vi "Set Control Value.vi"(8 "error in (no error)":errorcluster, 9 "value":variant, 11 "Panel":refnum<vi>) -> (0 "error out":errorcluster, 3 "Panel out":refnum<vi>)   [LabVIEW 2018, in "NISAST VI Scripting.lvlib" / "VI.lvlib" / "Front Panel.lvlib"]
uses:
  Front Panel.lvlib
  Type Define/Object Class.ctl
  Agilent N5232A PNA-L/Labview Driver/Keysight PNA Series/express/Utility/StudioHelper/Common/VI Scripting/Type Define/Type Define.lvlib
panel:
  in  "label":string
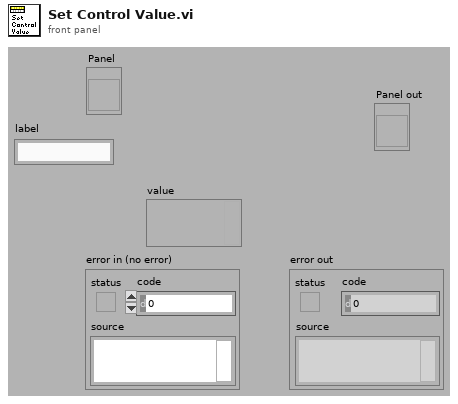
[diagram p1: front panel]
types:
  T1 = typedef "NISAST VI Scripting.lvlib/Type Define.lvlib/Object Class.ctl" = string
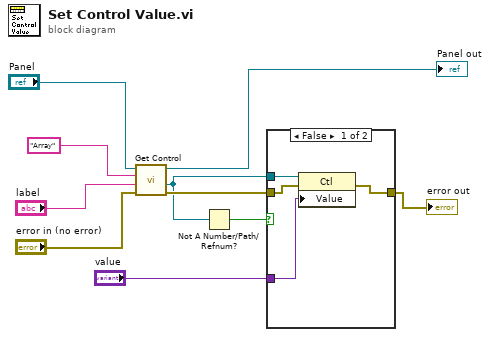
[diagram p0: block diagram]
diagram:
  n1 = call "Get Control.vi"("error in (no error)"="error in (no error)", "label"="label", "object class"=T1 "Array", "Panel"="Panel") -> ("error out"=w8:errorcluster, "first control"=w1:refnum<vi>, "Panel out"=→"Panel out":refnum<vi>)  [unwired: 5 out]
  n2 = Not A Number/Path/Refnum?(number/path/refnum=w1) -> (NaN/Path/Refnum?=w2:bool)
  n3 = case shown="False" w2 {
    tunnel: w1 -> [w14 _]
    tunnel: w8 -> [w13 w15]
    tunnel: "value" -> [w12 _]
    tunnel: [w11 w15] -> w5
    frame False {
      n4 = property class="Ctl"(reference=w14, error in=w13, "Value"=w12) -> (error out=w11:errorcluster)  [unwired: 1 out]
    }
    frame True {
    }
  }
  "error out" <- w5
